vi "Read LF2R Path.vi"(8 "error in (no error)":errorcluster) -> (0 "error out":errorcluster, 1 "PNG Path":path, 2 "Data Path":path, 3 "LF2R Path":path, 4 "Found":bool)   [LabVIEW 2018, in "LF2R IDE.lvlib" / "LF2R IDE.lvclass"]
uses:
  LF2R IDE.lvclass
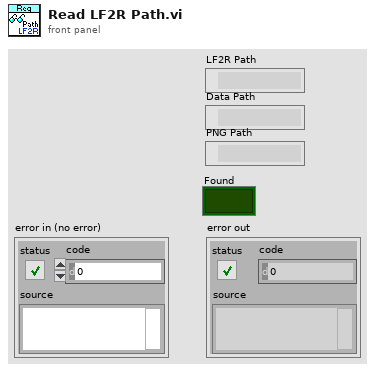
[diagram p1: front panel]
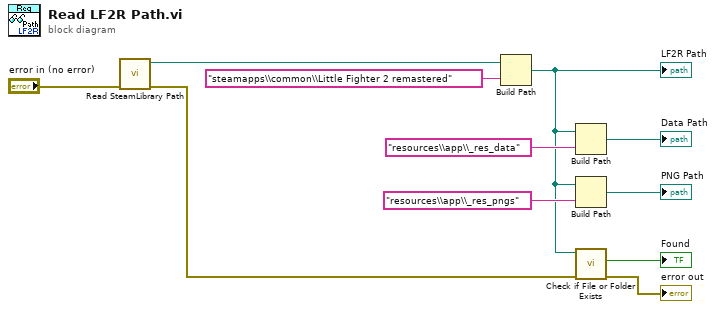
[diagram p0: block diagram]
diagram:
  n1 = call "Read SteamLibrary Path.vi"("error in (no error)"="error in (no error)") -> ("error out"=w1:errorcluster, "SteamLibrary Path"=w11:path)  [unwired: 8 in, 1 out]
  n2 = Build Path(base path=w11, name or relative path="steamapps\\common\\Little Fighter 2 remastered") -> (appended path=w4:path)
  "LF2R Path" <- w4
  n3 = Build Path(base path=w4, name or relative path="resources\\app\\_res_data") -> (appended path=→"Data Path":path)
  n4 = Build Path(base path=w4, name or relative path="resources\\app\\_res_pngs") -> (appended path=→"PNG Path":path)
  n5 = call <vilib>:"Check if File or Folder Exists.vi"("error in (no error)"=w1, "path"=w4) -> ("error out"=→"error out":errorcluster, "file or folder exists?"=→"Found":bool)  [unwired: 7 in, 1 out]
